vi "ABB Report remove fields.vi"(10 "Report in":string, 11 "Induction motor":bool) -> (2 "Report out":string)   [LabVIEW 2017]
uses:
  ABB global.vi
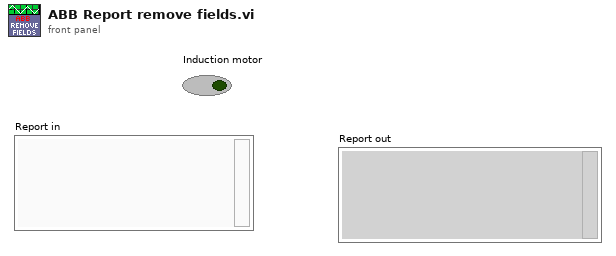
[diagram p1: front panel]
types:
  T1 = cluster{"temp. alloc":i32[], "category":i32[], "Category names":string[], "Category none names":string[]}
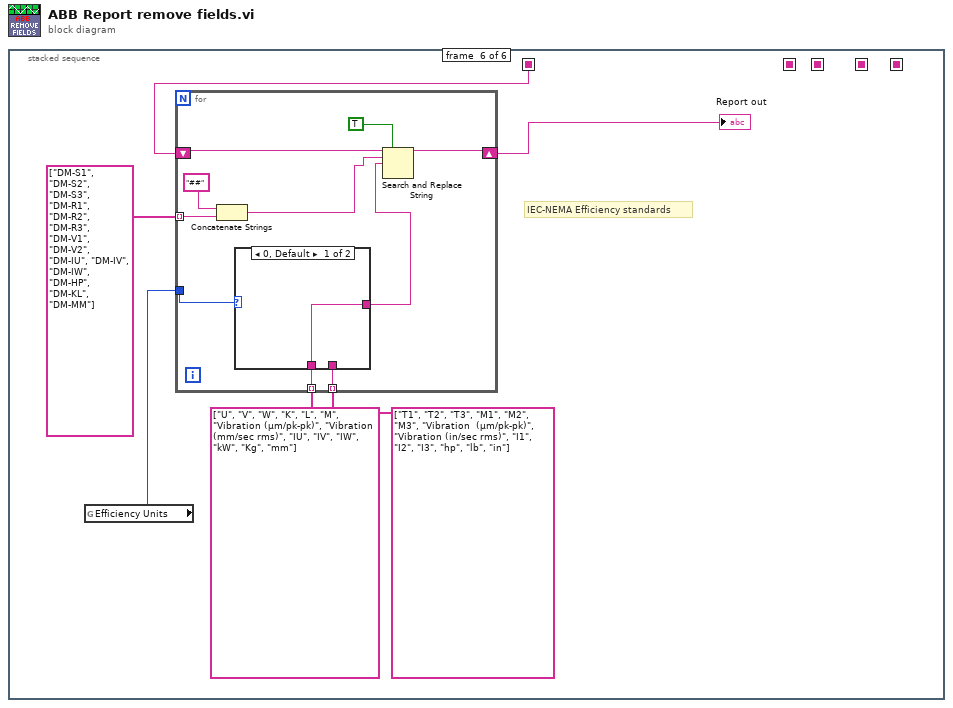
[diagram p0: block diagram]
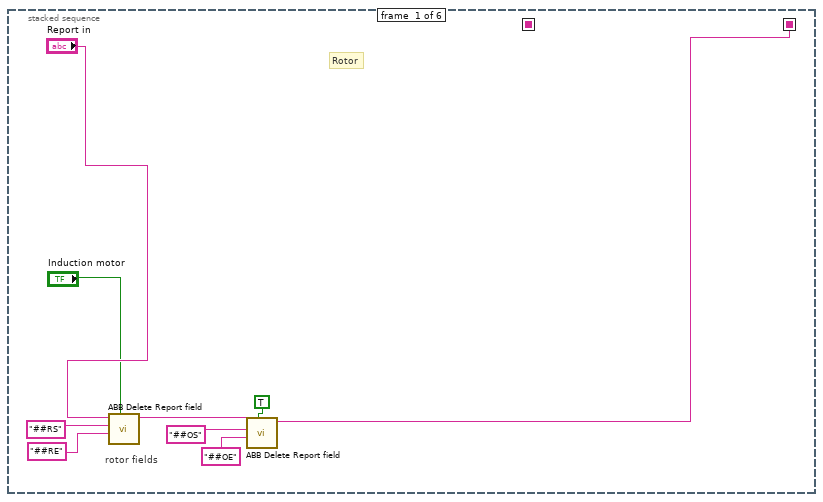
[diagram p2: hidden frame]
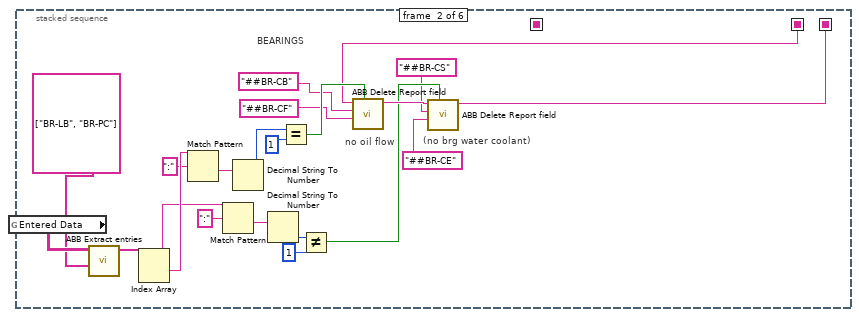
[diagram p3: hidden frame]
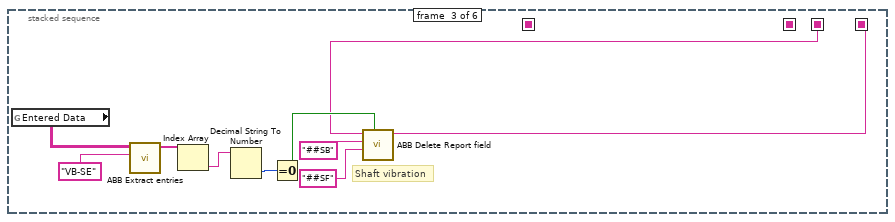
[diagram p4: hidden frame]
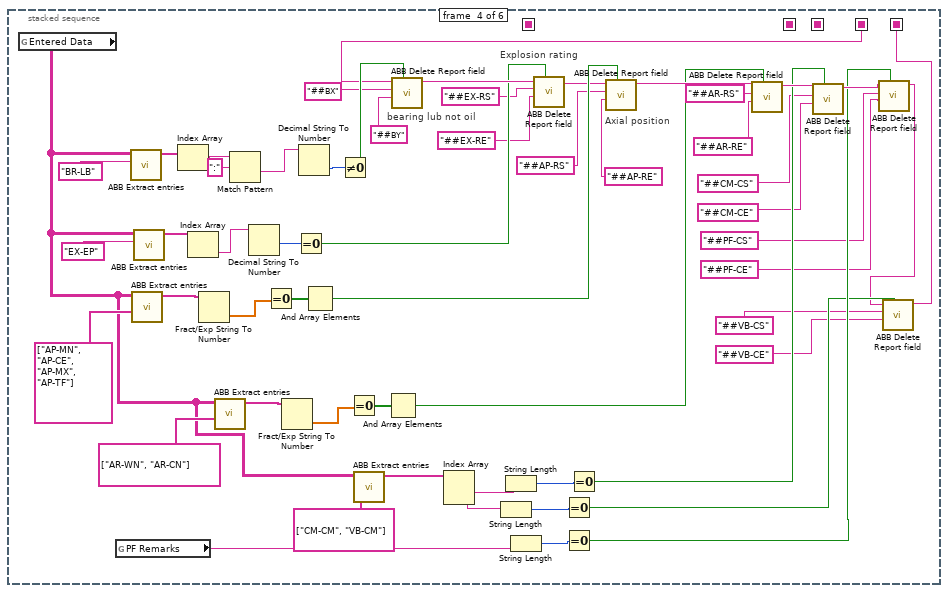
[diagram p5: hidden frame]
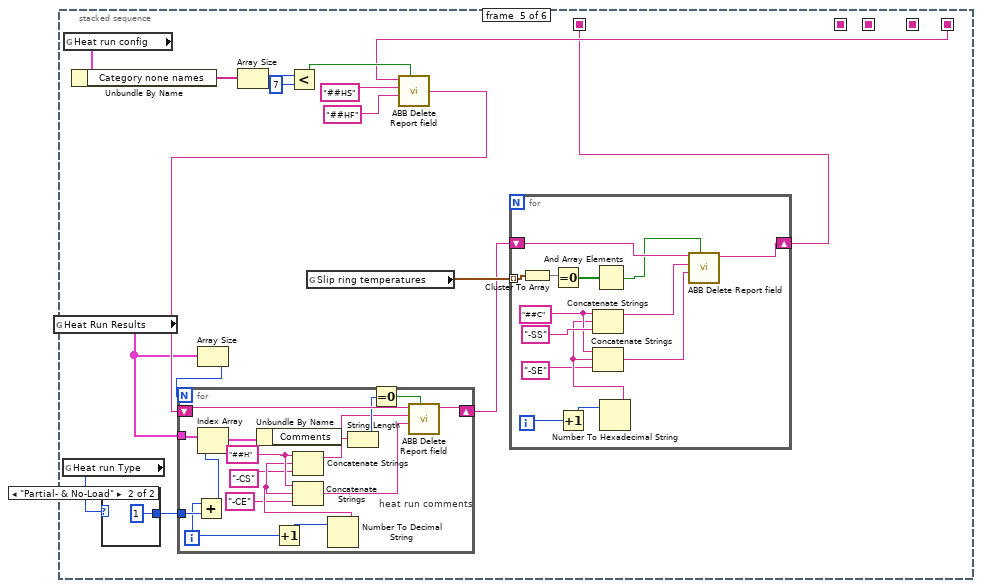
[diagram p6: hidden frame]
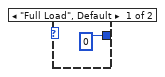
[diagram p7: hidden frame]
diagram:
  n1 = stacked-sequence {
    seq-local: [w9 _ _ _ _ _] -> [_ w15 _ _ _ _]
    seq-local: [_ _ w34 _ _ _] -> [_ _ _ w90 _ _]
    seq-local: [_ _ _ w44 _ _] -> [_ _ _ _ w108 _]
    seq-local: [_ w10 _ _ _ _] -> [_ _ w35 _ _ _]
    seq-local: [_ _ _ _ w98 _] -> [_ _ _ _ _ w150]
    frame #0 {
      # "rotor fields"
      # "Rotor"
      n2 = call "ABB Delete Report field.vi"("Delete"="Induction motor", "End"="##RE" ("regular expression"), "Start"="##RS" ("regular expression"), "Report in"="Report in") -> ("Report out"=w5:string)  [unwired: 7 in]
      n3 = call "ABB Delete Report field.vi"("Delete"=TRUE, "End"="##OE" ("regular expression"), "Start"="##OS" ("regular expression"), "Report in"=w5) -> ("Report out"=w9:string)  [unwired: 7 in]
    }
    frame #1 {
      # "BEARINGS"
      # "(no brg water coolant)"
      # "no oil flow"
      n4 = global read "ABB global.vi" "Entered Data"() -> (w31:string[][])
      n5 = call "ABB Extract entries.vi"("Entry IDs"=string[] ["BR-LB", "BR-PC"], "Entry table in"=w31) -> ("Selected Entries"=w29:string[])  [unwired: 9 in]
      n6 = Index Array(array=w29) -> (element #1=w28:string, element #2=w20:string)  [unwired: 2 in]
      n7 = Match Pattern(string=w28, regular expression=":") -> (after substring=w26:string)  [unwired: 1 in, 3 out]
      n8 = Match Pattern(string=w20, regular expression=":") -> (after substring=w23:string)  [unwired: 1 in, 3 out]
      n9 = Decimal String To Number(string=w26) -> (number=w25:i32)  [unwired: 2 in, 1 out]
      n10 = Decimal String To Number(string=w23) -> (number=w24:i32)  [unwired: 2 in, 1 out]
      n11 = Equal?(x=w25, y=1) -> (x = y?=w18:bool)
      n12 = Not Equal?(x=w24, y=1) -> (x != y?=w13:bool)
      n13 = call "ABB Delete Report field.vi"("Delete"=w18, "End"="##BR-CF" ("regular expression"), "Start"="##BR-CB" ("regular expression"), "Report in"=w15) -> ("Report out"=w14:string)  [unwired: 7 in]
      n14 = call "ABB Delete Report field.vi"("Delete"=w13, "End"="##BR-CE" ("regular expression"), "Start"="##BR-CS" ("regular expression"), "Report in"=w14) -> ("Report out"=w10:string)  [unwired: 7 in]
    }
    frame #2 {
      # "Shaft vibration"
      n15 = global read "ABB global.vi" "Entered Data"() -> (w41:string[][])
      n16 = call "ABB Extract entries.vi"("Entry ID"="VB-SE", "Entry table in"=w41) -> ("Selected Entries"=w39:string[])  [unwired: 9 in]
      n17 = Index Array(array=w39) -> (element=w38:string)  [unwired: 1 in]
      n18 = Decimal String To Number(string=w38) -> (number=w37:i32)  [unwired: 2 in, 1 out]
      n19 = Equal To 0?(x=w37) -> (x = 0?=w36:bool)
      n20 = call "ABB Delete Report field.vi"("Delete"=w36, "End"="##SF" ("regular expression"), "Start"="##SB" ("regular expression"), "Report in"=w35) -> ("Report out"=w34:string)  [unwired: 7 in]
    }
    frame #3 {
      # "Axial position"
      # "Explosion rating"
      # "bearing lub not oil"
      n21 = global read "ABB global.vi" "Entered Data"() -> (w63:string[][])
      n22 = global read "ABB global.vi" "PF Remarks"() -> (w49:string)
      n23 = call "ABB Extract entries.vi"("Entry ID"="BR-LB", "Entry table in"=w63) -> ("Selected Entries"=w96:string[])  [unwired: 9 in]
      n24 = call "ABB Extract entries.vi"("Entry IDs"=string[] ["AP-MN", "AP-CE", "AP-MX", "AP-TF"], "Entry table in"=w63) -> ("Selected Entries"=w78:string[])  [unwired: 9 in]
      n25 = call "ABB Extract entries.vi"("Entry ID"="EX-EP", "Entry table in"=w63) -> ("Selected Entries"=w86:string[])  [unwired: 9 in]
      n26 = Index Array(array=w96) -> (element=w94:string)  [unwired: 1 in]
      n27 = Index Array(array=w86) -> (element=w85:string)  [unwired: 1 in]
      n28 = Fract/Exp String To Number(string=w78) -> (number=w77:dbl[])  [unwired: 3 in, 1 out]
      n29 = call "ABB Extract entries.vi"("Entry IDs"=string[] ["AR-WN", "AR-CN"], "Entry table in"=w63) -> ("Selected Entries"=w69:string[])  [unwired: 9 in]
      n30 = Match Pattern(string=w94, regular expression=":") -> (after substring=w92:string)  [unwired: 1 in, 3 out]
      n31 = Decimal String To Number(string=w85) -> (number=w84:i32)  [unwired: 2 in, 1 out]
      n32 = Equal To 0?(x=w77) -> (x = 0?=w76:bool[])
      n33 = Fract/Exp String To Number(string=w69) -> (number=w70:dbl[])  [unwired: 3 in, 1 out]
      n34 = Equal To 0?(x=w84) -> (x = 0?=w82:bool)
      n35 = Decimal String To Number(string=w92) -> (number=w95:i32)  [unwired: 2 in, 1 out]
      n36 = And Array Elements(Boolean array=w76) -> (logical AND=w75:bool)
      n37 = Not Equal To 0?(x=w95) -> (x != 0?=w91:bool)
      n38 = Equal To 0?(x=w70) -> (x = 0?=w71:bool[])
      n39 = call "ABB Extract entries.vi"("Entry IDs"=string[] ["CM-CM", "VB-CM"], "Entry table in"=w63) -> ("Selected Entries"=w61:string[])  [unwired: 9 in]
      n40 = And Array Elements(Boolean array=w71) -> (logical AND=w66:bool)
      n41 = call "ABB Delete Report field.vi"("Delete"=w91, "End"="##BY" ("search string"), "Start"="##BX" ("regular expression"), "Report in"=w90) -> ("Report out"=w83:string)  [unwired: 7 in]
      n42 = Index Array(array=w61) -> (element #1=w60:string, element #2=w47:string)  [unwired: 2 in]
      n43 = String Length(string=w47) -> (length=w48:i32)
      n44 = String Length(string=w60) -> (length=w59:i32)
      n45 = String Length(string=w49) -> (length=w54:i32)
      n46 = call "ABB Delete Report field.vi"("Delete"=w82, "End"="##EX-RE" ("search string"), "Start"="##EX-RS" ("regular expression"), "Report in"=w83) -> ("Report out"=w74:string)  [unwired: 7 in]
      n47 = Equal To 0?(x=w48) -> (x = 0?=w46:bool)
      n48 = Equal To 0?(x=w54) -> (x = 0?=w52:bool)
      n49 = Equal To 0?(x=w59) -> (x = 0?=w57:bool)
      n50 = call "ABB Delete Report field.vi"("Delete"=w75, "End"="##AP-RE", "Start"="##AP-RS", "Report in"=w74) -> ("Report out"=w67:string)  [unwired: 7 in]
      n51 = call "ABB Delete Report field.vi"("Delete"=w66, "End"="##AR-RE", "Start"="##AR-RS", "Report in"=w67) -> ("Report out"=w58:string)  [unwired: 7 in]
      n52 = call "ABB Delete Report field.vi"("Delete"=w57, "End"="##CM-CE" ("Start"), "Start"="##CM-CS", "Report in"=w58) -> ("Report out"=w53:string)  [unwired: 7 in]
      n53 = call "ABB Delete Report field.vi"("Delete"=w52, "End"="##PF-CE" ("Start"), "Start"="##PF-CS", "Report in"=w53) -> ("Report out"=w45:string)  [unwired: 7 in]
      n54 = call "ABB Delete Report field.vi"("Delete"=w46, "End"="##VB-CE" ("Start"), "Start"="##VB-CS", "Report in"=w45) -> ("Report out"=w44:string)  [unwired: 7 in]
    }
    frame #4 {
      n55 = global read "ABB global.vi" "Heat Run Results"() -> (w100:cluster{"results":dbl[][], "Comments":string}[])
      n56 = global read "ABB global.vi" "Heat run Type"() -> (w102:enum16{"Full Load", "Partial- & No-Load"})
      n57 = global read "ABB global.vi" "Heat run config"() -> (w113:T1)
      n58 = Unbundle By Name(w113) -> ("Category none names"=w112:string[])
      n59 = case shown="\"Partial- & No-Load\"" w102 {
        tunnel: [0 1] -> w101
        frame "Full Load", Default {
        }
        frame "Partial- & No-Load" {
        }
      }
      n60 = Array Size(array=w100) -> (size(s)=w99:i32)
      n61 = Array Size(array=w112) -> (size(s)=w111:i32)
      n62 = Less?(x=w111, y=7) -> (x < y?=w109:bool)
      n63 = global read "ABB global.vi" "Slip ring temperatures"() -> (w105:cluster{"K":dbl, "L":dbl, "M ":dbl}[])
      n64 = call "ABB Delete Report field.vi"("Delete"=w109, "End"="##HF" ("regular expression"), "Start"="##HS" ("regular expression"), "Report in"=w108) -> ("Report out"=w104:string)  [unwired: 7 in]
      n65 = for {
        N: w99 -> [_]
        tunnel: w100 -> [w120]
        shift-right: [w121] -> w103
        shift-left: w104 -> [w126]
        tunnel: w101 -> [w118]
        i -> [w117]
        w130 = "##H" ("string")
        # "heat run comments"
        n66 = Add(x=w117, y=w118) -> (x+y=w116:i32)
        n67 = Index Array(array=w120, index=w116) -> (element=w119:cluster{"results":dbl[][], "Comments":string})
        n68 = Unbundle By Name(w119) -> ("Comments"=w132:string)
        n69 = Increment(x=w117) -> (x+1=w131:i32)
        n70 = Number To Decimal String(number=w131) -> (decimal integer string=w129:string)  [unwired: 1 in]
        n71 = Concatenate Strings(w130, w129, "-CS") -> (w123:string)
        n72 = Concatenate Strings(w130, w129, "-CE" ("string")) -> (w122:string)
        n73 = String Length(string=w132) -> (length=w125:i32)
        n74 = Equal To 0?(x=w125) -> (x = 0?=w124:bool)
        n75 = call "ABB Delete Report field.vi"("Delete"=w124, "End"=w122, "Start"=w123, "Report in"=w126) -> ("Report out"=w121:string)  [unwired: 7 in]
      }
      n76 = for {
        shift-right: [w142] -> w98
        shift-left: w103 -> [w143]
        tunnel: w105 -> [w146] mode=indexing
        i -> [w141]
        w138 = "##C"
        n77 = Cluster To Array(cluster=w146) -> (array=w145:dbl[])
        n78 = Equal To 0?(x=w145) -> (x = 0?=w144:bool[])
        n79 = Increment(x=w141) -> (x+1=w140:i32)
        n80 = And Array Elements(Boolean array=w144) -> (logical AND=w133:bool)
        n81 = Number To Hexadecimal String(2:w140) -> (0:w137:string)  [unwired: 1 in]
        n82 = Concatenate Strings(w138, w137, "-SS" ("string")) -> (w135:string)
        n83 = Concatenate Strings(w138, w137, "-SE" ("string")) -> (w134:string)
        n84 = call "ABB Delete Report field.vi"("Delete"=w133, "End"=w134, "Start"=w135, "Report in"=w143) -> ("Report out"=w142:string)  [unwired: 7 in]
      }
    }
    frame #5 {
      # "IEC-NEMA Efficiency standards"
      n85 = global read "ABB global.vi" "Efficiency Units"() -> (w151:u16)
      n86 = for {
        tunnel: string[] ["DM-S1", "DM-S2", "DM-S3", "DM-R1", "DM-R2", "DM-R3", "DM-V1", "DM-V2", "DM-IU", "DM-IV", "DM-IW", "DM-HP", "DM-KL", "DM-MM"] -> [w160] mode=indexing
        tunnel: w151 -> [w157]
        shift-right: [w161] -> w148
        shift-left: w150 -> [w162]
        tunnel: string[] ["U", "V", "W", "K", "L", "M", "Vibration (µm/pk-pk)", "Vibration (mm/sec rms)", "IU", "IV", "IW", "kW", "Kg", "mm"] -> [w156] mode=indexing
        tunnel: string[] ["T1", "T2", "T3", "M1", "M2", "M3", "Vibration  (µm/pk-pk)", "Vibration (in/sec rms)", "I1", "I2", "I3", "hp", "lb", "in"] -> [w153] mode=indexing
        n87 = Concatenate Strings("##", w160) -> (w158:string)
        n88 = case shown="0, Default" w157 {
          tunnel: w156 -> [w163 _]
          tunnel: [w163 w164] -> w155
          tunnel: w153 -> [_ w164]
          frame 0, Default {
          }
          frame 1 {
          }
        }
        n89 = Search and Replace String(replace all?=TRUE ("replace all? (F)"), input string=w162, search string=w158, replace string=w155) -> (result string=w161:string)  [unwired: 4 in, 3 out]
      }
      "Report out" <- w148
    }
  }
